vi "p12.vi"() -> ()   [LabVIEW 2015]
panel:
  out "Invert ADD":dbl[](array[numeric])
  out "Invert MUL":dbl[](array[numeric])
  out "Numeric : Compound AND":dbl
  out "No. --> Array":bool[](array[boolean])
  out "Array --> No.":u32
  out "logical AND":bool
  out "logical OR":bool
  out "0, 1":i16[](array[numeric])
  out "Array : Compound AND":bool[](array[boolean])
  out "Compound AND":bool
  out "Binary IMPLIES":i8 format="%08b"
  out "Binary AND":i32 format="%08b"
  out "Numeric IMPLIES":i32
  out "Boolean IMPLIES":bool
  out "Error Cluster IMPLIES":bool
  out "Numeric EX-OR":i32
  out "Boolean EX-OR":bool
  out "Error Cluster EX-OR":bool
  out "Numeric OR":i32
  out "Boolean OR":bool
  out "Error Cluster OR":bool
  out "Numeric AND":i32
  out "Boolean AND":bool
  out "Error Cluster AND":bool
  # "AND OPERATOR"
  # "AND OPERATOR"
  # "AND OPERATOR"
  # "AND OPERATOR"
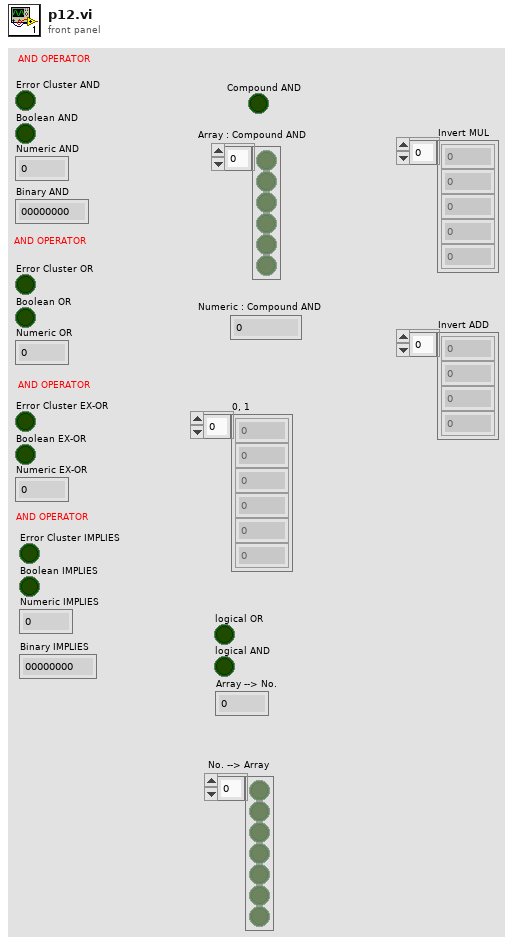
[diagram p1: front panel]
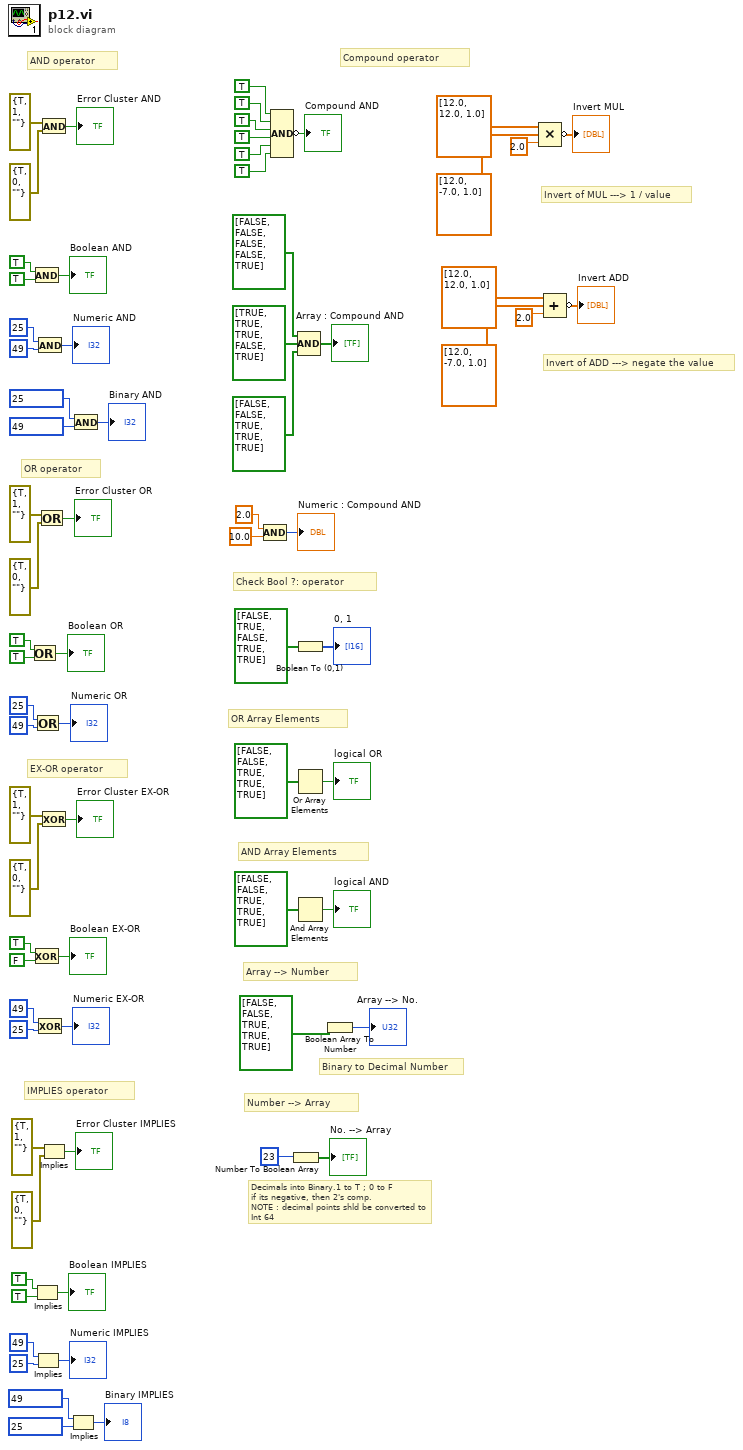
[diagram p0: block diagram]
diagram:
  # "Invert of ADD ---> negate the value"
  # "Invert of MUL ---> 1 / value"
  # "Decimals into Binary.1 to T ; 0 to F\nif its negative, then 2's comp.\nNOTE : decimal points shld be converted to Int 64"
  # "Number --> Array"
  # "Binary to Decimal Number"
  # "Array --> Number"
  # "AND Array Elements"
  # "OR Array Elements"
  # "Check Bool ?: operator"
  # "Compound operator"
  # "IMPLIES operator"
  # "EX-OR operator"
  # "OR operator"
  # "AND operator"
  n1 = Or(x=TRUE, y=TRUE ("x")) -> (x .or. y?=→"Boolean OR":bool)
  n2 = And(x=TRUE, y=TRUE ("x")) -> (x .and. y?=→"Boolean AND":bool)
  n3 = Exclusive Or(1:FALSE ("x"), 2:TRUE ("x")) -> (0:→"Boolean EX-OR":bool)
  n4 = Implies(1:TRUE ("x"), 2:TRUE ("x")) -> (0:→"Boolean IMPLIES":bool)
  n5 = Or(x=25, y=49) -> (x .or. y?=→"Numeric OR":i32)
  n6 = Implies(1:25, 2:49) -> (0:→"Numeric IMPLIES":i32)
  n7 = And(x=25, y=49) -> (x .and. y?=→"Numeric AND":i32)
  n8 = Exclusive Or(1:25, 2:49) -> (0:→"Numeric EX-OR":i32)
  n9 = Or(x=errorcluster {"status"=TRUE, "code"=1, "source"=""} ("error constant"), y=errorcluster {"status"=TRUE, "code"=0, "source"=""} ("error constant")) -> (x .or. y?=→"Error Cluster OR":bool)
  n10 = And(x=errorcluster {"status"=TRUE, "code"=1, "source"=""} ("error constant"), y=errorcluster {"status"=TRUE, "code"=0, "source"=""} ("error constant")) -> (x .and. y?=→"Error Cluster AND":bool)
  n11 = Exclusive Or(1:errorcluster {"status"=TRUE, "code"=0, "source"=""} ("error constant"), 2:errorcluster {"status"=TRUE, "code"=1, "source"=""} ("error constant")) -> (0:→"Error Cluster EX-OR":bool)
  n12 = Implies(1:errorcluster {"status"=TRUE, "code"=0, "source"=""} ("error constant"), 2:errorcluster {"status"=TRUE, "code"=1, "source"=""} ("error constant")) -> (0:→"Error Cluster IMPLIES":bool)
  n13 = Implies(1:i8 25, 2:i8 49) -> (0:→"Binary IMPLIES":i8)
  n14 = And(x=25, y=49) -> (x .and. y?=→"Binary AND":i32)
  n15 = Compound Arithmetic op=AND(2.0 ("value"), 10.0 ("value")) -> (→"Numeric : Compound AND":i32)
  n16 = Compound Arithmetic op=AND(TRUE ("x"), TRUE ("x"), TRUE ("x"), TRUE ("x"), TRUE ("x"), TRUE ("x")) -> (invert →"Compound AND":bool)
  n17 = Number To Boolean Array(number=i64 23) -> (Boolean array=→"No. --> Array":bool[])
  n18 = Boolean To (0,1)(Boolean=bool[] [FALSE, TRUE, FALSE, TRUE, TRUE]) -> (0, 1=→"0, 1":i16[])
  n19 = Or Array Elements(Boolean array=bool[] [FALSE, FALSE, TRUE, TRUE, TRUE]) -> (logical OR=→"logical OR":bool)
  n20 = And Array Elements(Boolean array=bool[] [FALSE, FALSE, TRUE, TRUE, TRUE]) -> (logical AND=→"logical AND":bool)
  n21 = Compound Arithmetic op=AND(bool[] [FALSE, FALSE, FALSE, FALSE, TRUE], bool[] [TRUE, TRUE, TRUE, FALSE, TRUE], bool[] [FALSE, FALSE, TRUE, TRUE, TRUE]) -> (→"Array : Compound AND":bool[])
  n22 = Boolean Array To Number(Boolean array=bool[] [FALSE, FALSE, TRUE, TRUE, TRUE]) -> (number=→"Array --> No.":u32)
  n23 = Compound Arithmetic op=MULTIPLY(dbl[] [12.0, 12.0, 1.0], dbl[] [12.0, -7.0, 1.0], 2.0 ("value")) -> (invert →"Invert MUL":dbl[])
  n24 = Compound Arithmetic op=unknown(dbl[] [12.0, 12.0, 1.0], dbl[] [12.0, -7.0, 1.0], 2.0 ("value")) -> (invert →"Invert ADD":dbl[])
